vi "GBL DataQ Refs.vi"() -> ()   [LabVIEW 2022 SP3, in "DAQ.lvclass"]
doc: "Developed by Kevin Thompson\nkevin@thompsonengineering.net\n\nCopyright 2018-2020\nThompson Engineering, LLC"
uses:
  DAQ.lvclass
panel:
  in  "DAQ PrimeTimer QRef":u32
  in  "DAQ eTime QRef":u32
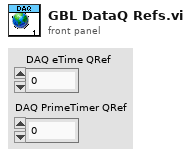
[diagram p1: front panel]
diagram:
